vi "Robot Global Data.vi"() -> ()   [LabVIEW 2013]
doc: "This global VI can contain as many global variables as you need. Place a control on the panel, give it a good name. To read or write to it from a VI, drag the icon to the diagram of that VI. You can also drag from the project. Click on the node to change which global you access. You shouldn't have multiple locations writing to a global or it will cause a race-condition."
uses:
  <vilib>/Rock Robotics/WPI/DriverStation/WPI_DriverStationRobotMode2.ctl
  Drivetrain/Drivetrain Control.ctl
  Drivetrain/DT Mode.ctl
  Rollers/Roller Control.ctl
  Rollers/Roller Mode.ctl
  Common Code/Vision Packet.ctl
  Common Code/Goal Info.ctl
  Drivetrain/Arcade Drive Ref.ctl
  <vilib>/Rock Robotics/WPI/MotorControl/WPI_MotorControlDeviceRef.ctl
  <vilib>/Rock Robotics/SystemInterfaces/Typedef/FPGA_TypedefDigitalModule.ctl
  <vilib>/Rock Robotics/SystemInterfaces/DIO/FPGA_DIOPWMChannel.ctl
  <vilib>/Rock Robotics/WPI/PWM/WPI_PWMDeadband.ctl
  <vilib>/Rock Robotics/WPI/CAN/Jaguar/SubVIs/WPI_CANJaguar_ControlMode.ctl
  <vilib>/Rock Robotics/WPI/PWM/WPI_PWMTransform_ConPane.ctl
  Shooter/Shooter Manual Control.ctl
  Shooter/Shooter Command.ctl
  Drivetrain/Distance Drive Result.ctl
  Common Code/Dashboard UDP Packet.ctl
  Common Code/Dashboard UDP/Camera Controls.ctl
  Common Code/Dashboard UDP/Gyro Controls.ctl
  Common Code/Dashboard UDP/PID Params.ctl
  Common Code/Dashboard UDP/Encoder Controls.ctl
  Common Code/Dashboard UDP/Auto Shift Controls.ctl
  Common Code/Dashboard UDP/Auton Controls.ctl
  Common Code/Dashboard UDP/Shooter Controls.ctl
  Common Code/Dashboard UDP/Roller Controls.ctl
  Common Code/Vision Mode.ctl
  Common Code/Dashboard UDP/Fieldcentric Controls.ctl
  Common Code/Dashboard UDP/Roll Maneuver.ctl
  Drivetrain/Drivetrain Status.ctl
  Rollers/Roller Status.ctl
  Common Code/IR Logic State.ctl
  Shooter/Shooter Status.ctl
  Common Code/Shooter State.ctl
panel:
  out "Auton Enabled Time":u32
  out "Invert Halo":bool
  out "Halo Up Time":i32
  out "Halo":bool
  out "Manual Halo":bool
  out "Auto Halo":bool
  out "Shooter Wants Halo":bool
  out "Roller Wants Halo":bool
  out "100ms Loop Time":i32
  out "Auton File Display":string
  out "Auton Command Count":i32
  out "Auton Command":i32
  out "Shooter Status":T1
  out "Roller Status":T3
  out "Gyro Target":dbl
  out "Drivetrain Status":T5
  in  "Auton File":dbl
  out "UDP Packet":T7={"Camera"={"Camera/View Angle X"=66.5, "Camera/Goal Track Timeout"=120.0, "Camera/View Angle Y"=49.0, "Camera/Goal Exposure"=0.0, "Camera/Vision Receive Timeout"=120.0, "Camera/Offset 1"=-35.0, "Camera/Offset 2"=35.0}, "Gyro"={"Gyro/Angle Tolerance"=2.0, "Gyro/Steer Closeness Threshold"=10.0, "Steer PID"={"max"=0.8, "min"=-0.8, "P"=0.04, "I"=0.0, "D"=0.0}, "Steer Close PID"={"max"=0.7, "min"=-0.7, "P"=0.04, "I"=0.0, "D"=0.002}}, "Encoder"={"Encoders/Reset"=FALSE, "Encoders/Omni Constant"=0.002909, "Encoders/Omni Tick Constant"=1.0, "Encoders/Left Constant"=0.000546, "Encoders/Right Constant"=0.000546, "Encoders/Right Tick Constant"=1.0}, "Auto Shift"={"AutoShift/Upshift Throttle Accel"=-2.0, "AutoShift/Speed Threshold"=5.0, "AutoShift/Upshift Throttle"=0.8, "AutoShift/Upshift Accel"=0.5, "AutoShift/Downshift Accel"=-1.2, "AutoShift/Downshift Throttle"=0.15, "AutoShift/Delay"=1000.0, "AutoShift/Enabled"=TRUE}, "Auton"={"Auton/Left Shoot X-Coord"=-4.0, "Auton/Right Shoot X-Coord"=4.0, "DistDrive/Distance Stop Threshold"=0.25, "DistDrive/Max Stop Speed"=0.5, "Auton/Back Piston Time"=500.0, "Auton/Manual Hot"=FALSE, "Auton/Manual Hot Right"=FALSE, "Default X PID"={"max"=1.0, "min"=-1.0, "P"=0.36, "I"=0.0, "D"=0.0}, "Default Y PID"={"max"=1.0, "min"=-1.0, "P"=0.7, "I"=0.0, "D"=0.001}, "Half Over Delay"=4500.0}, "Drive/Ramp X"=500.0, "Drive/Ramp Y"=250.0, "Drive/Battery Cutoff"=6.0, "Pressure/Compressor Min Voltage"=7.0, "Pressure/Compressor Delay"=500.0, "Controller/Strafe Correction"=TRUE, "Shooter"={"Shooter/Reset Time"=500.0, "Shooter/Release Delay"=150.0, "Shooter/Pressure Steady Time"=0.0, "Shooter/Misfire Delay"=2000.0, "Shooter/Ball Settle Time"=500.0, "Shooter/Line IR Delay"=300.0, "Pressure/Upper PSI Time"=500.0, "Pressure/Lower PSI Time"=500.0, "Shooter/Punch Delay"=-150.0, "Shooter/Target Pressure"=43.0, "Pressure/Line B"=-57.077, "Pressure/Line M"=33.41, "Pressure/Shooter M"=33.41, "Pressure/Shooter B"=-57.077, "Halo Time"=150.0, "Soft Release Delay"=800.0, "Soft Unpin Delay"=250.0, "Soft Shoot Delay"=290.0, "Toss Release Time"=62.4}, "Rollers"={"Roller/Load IRs Verify Time"=150.0, "Roller/Center IR Latch Time"=500.0, "Roller/Speed Front"=1.0, "Roller/Speed Back"=0.6, "Roller/Entry Timeout"=750.0, "Roller/To Center Timeout"=2000.0, "Roller/Sustain Time"=5000.0, "Roller/Verify Center Time"=250.0}, "Abort"=FALSE, "Finish"=FALSE, "IR Halo Sustain Time"=0.0, "Disable Compressor"=FALSE, "Center Omni Drive Delay"=100, "Vision Mode"=enum."Normal", "Radius Throttle"=TRUE, "Fieldcentric"={"Relative Angle"=TRUE, "Point Robot"=FALSE, "X/Y ratio low"=0.75, "Steering Gain"=1.0, "Force Omni Down"=TRUE, "Enable"=TRUE, "X/Y ratio high"=0.5}, "Roll"={"X 1"=0.0, "Y 1"=1.0, "Y 2"=1.0, "X 2"=1.0, "Y 3"=1.0, "X 3"=0.0, "Time 1"=300, "Time 2"=1000, "Time 3"=0, "Angle Start"=0.0, "Angle End"=-180.0, "Angle Linearity"=1.0}, "Stick Deadband"=0.075}
  out "Distance Drive Result":T19
  out "Robot Direction":enum16{"Forward", "Backward"}(ring)
  out "Robot Orientation":enum16{"Away", "Towards"}(ring)
  out "LineJustCrossed":enum16{"None", "Blue", "Red"}(ring)
  out "Zone":enum16{"Blue", "White", "Red"}(ring)=enum."Red"
  out "Line Crossed?":bool
  out "Line Heading Towards":enum16{"Red", "Blue"}(ring)
  out "Last Shoot Begin Time":u32
  out "Goals Used":i32
  out "Hot Found":bool
  out "Shoot High Pressure":bool
  in  "Interrupt Negated":bool
  in  "Finish":bool
  in  "Abort":bool
  in  "Interrupt Condition":i32
  in  "Interrupt Index":i32
  in  "Interrupt Set":bool
  out "Gyro Calibrating":bool
  out "Recalibrate Gyro":refnum<k4>
  out "Last Shoot Time":u32
  out "Camera 2 Packet":T20
  out "Camera 2 Connected":bool
  out "Camera 1 Connected":bool
  in  "Shooter Control":T22
  out "Gyro in Range":bool
  in  "Roller Control":T24
  out "Find Ball?":bool
  in  "isQuietRun":bool
  out "isRightHot":bool
  out "Cam Search Enabled":bool
  in  "Vision UDP Connection":refnum<k16>
  in  "Selection controls":cluster{"Up":bool, "Down":bool}
  in  "FilesInAutonDir":i32
  out "Camera 1 Packet":T20
  out "Auto Array":dbl[][](array[numeric]) format="%0.3f"
  in  "Drivetrain Control":T26={"axis 1 (x)"=0.0, "axis 2 (y)"=0.0, "Mode"=enum."Manual", "heading target"=0.0, "steer axis"=0.0, "omni?"=FALSE, "Low Gear?"=FALSE, "distance target"={"x"=0.0, "y"=0.0}, "PID Params"={"X Dist"={"PID gains"={"proportional gain (Kc)"=1.0, "integral time (Ti, min)"=0.0, "derivative time (Td, min)"=0.0}, "output range"={"output high"=1.0, "output low"=-1.0}}, "Y Dist"={"PID gains"={"proportional gain (Kc)"=1.0, "integral time (Ti, min)"=0.0, "derivative time (Td, min)"=0.0}, "output range"={"output high"=1.0, "output low"=-1.0}}}, "Coast"=FALSE} {"PID Params"."Y Dist"."output range"."output low" format="%.2f"; "PID Params"."Y Dist"."output range"."output high" format="%.2f"; "PID Params"."Y Dist"."PID gains"."derivative time (Td, min)" format="%.3f"; "PID Params"."Y Dist"."PID gains"."integral time (Ti, min)" format="%.3f"; "PID Params"."Y Dist"."PID gains"."proportional gain (Kc)" format="%.3f"; "PID Params"."X Dist"."output range"."output low" format="%.2f"; "PID Params"."X Dist"."output range"."output high" format="%.2f"; "PID Params"."X Dist"."PID gains"."derivative time (Td, min)" format="%.3f"; "PID Params"."X Dist"."PID gains"."integral time (Ti, min)" format="%.3f"; "PID Params"."X Dist"."PID gains"."proportional gain (Kc)" format="%.3f"}
  in  "Robot Mode":T27
  out "Arcade Drive":T28
  # "Note: default values here are meaningless,\nSet default values in \"Load Preferences.vi\""
  # "Autonomous Stuff"
  # "Line"
  # "Shooter"
  # "Down"
  # "Up"
  # "Feet"
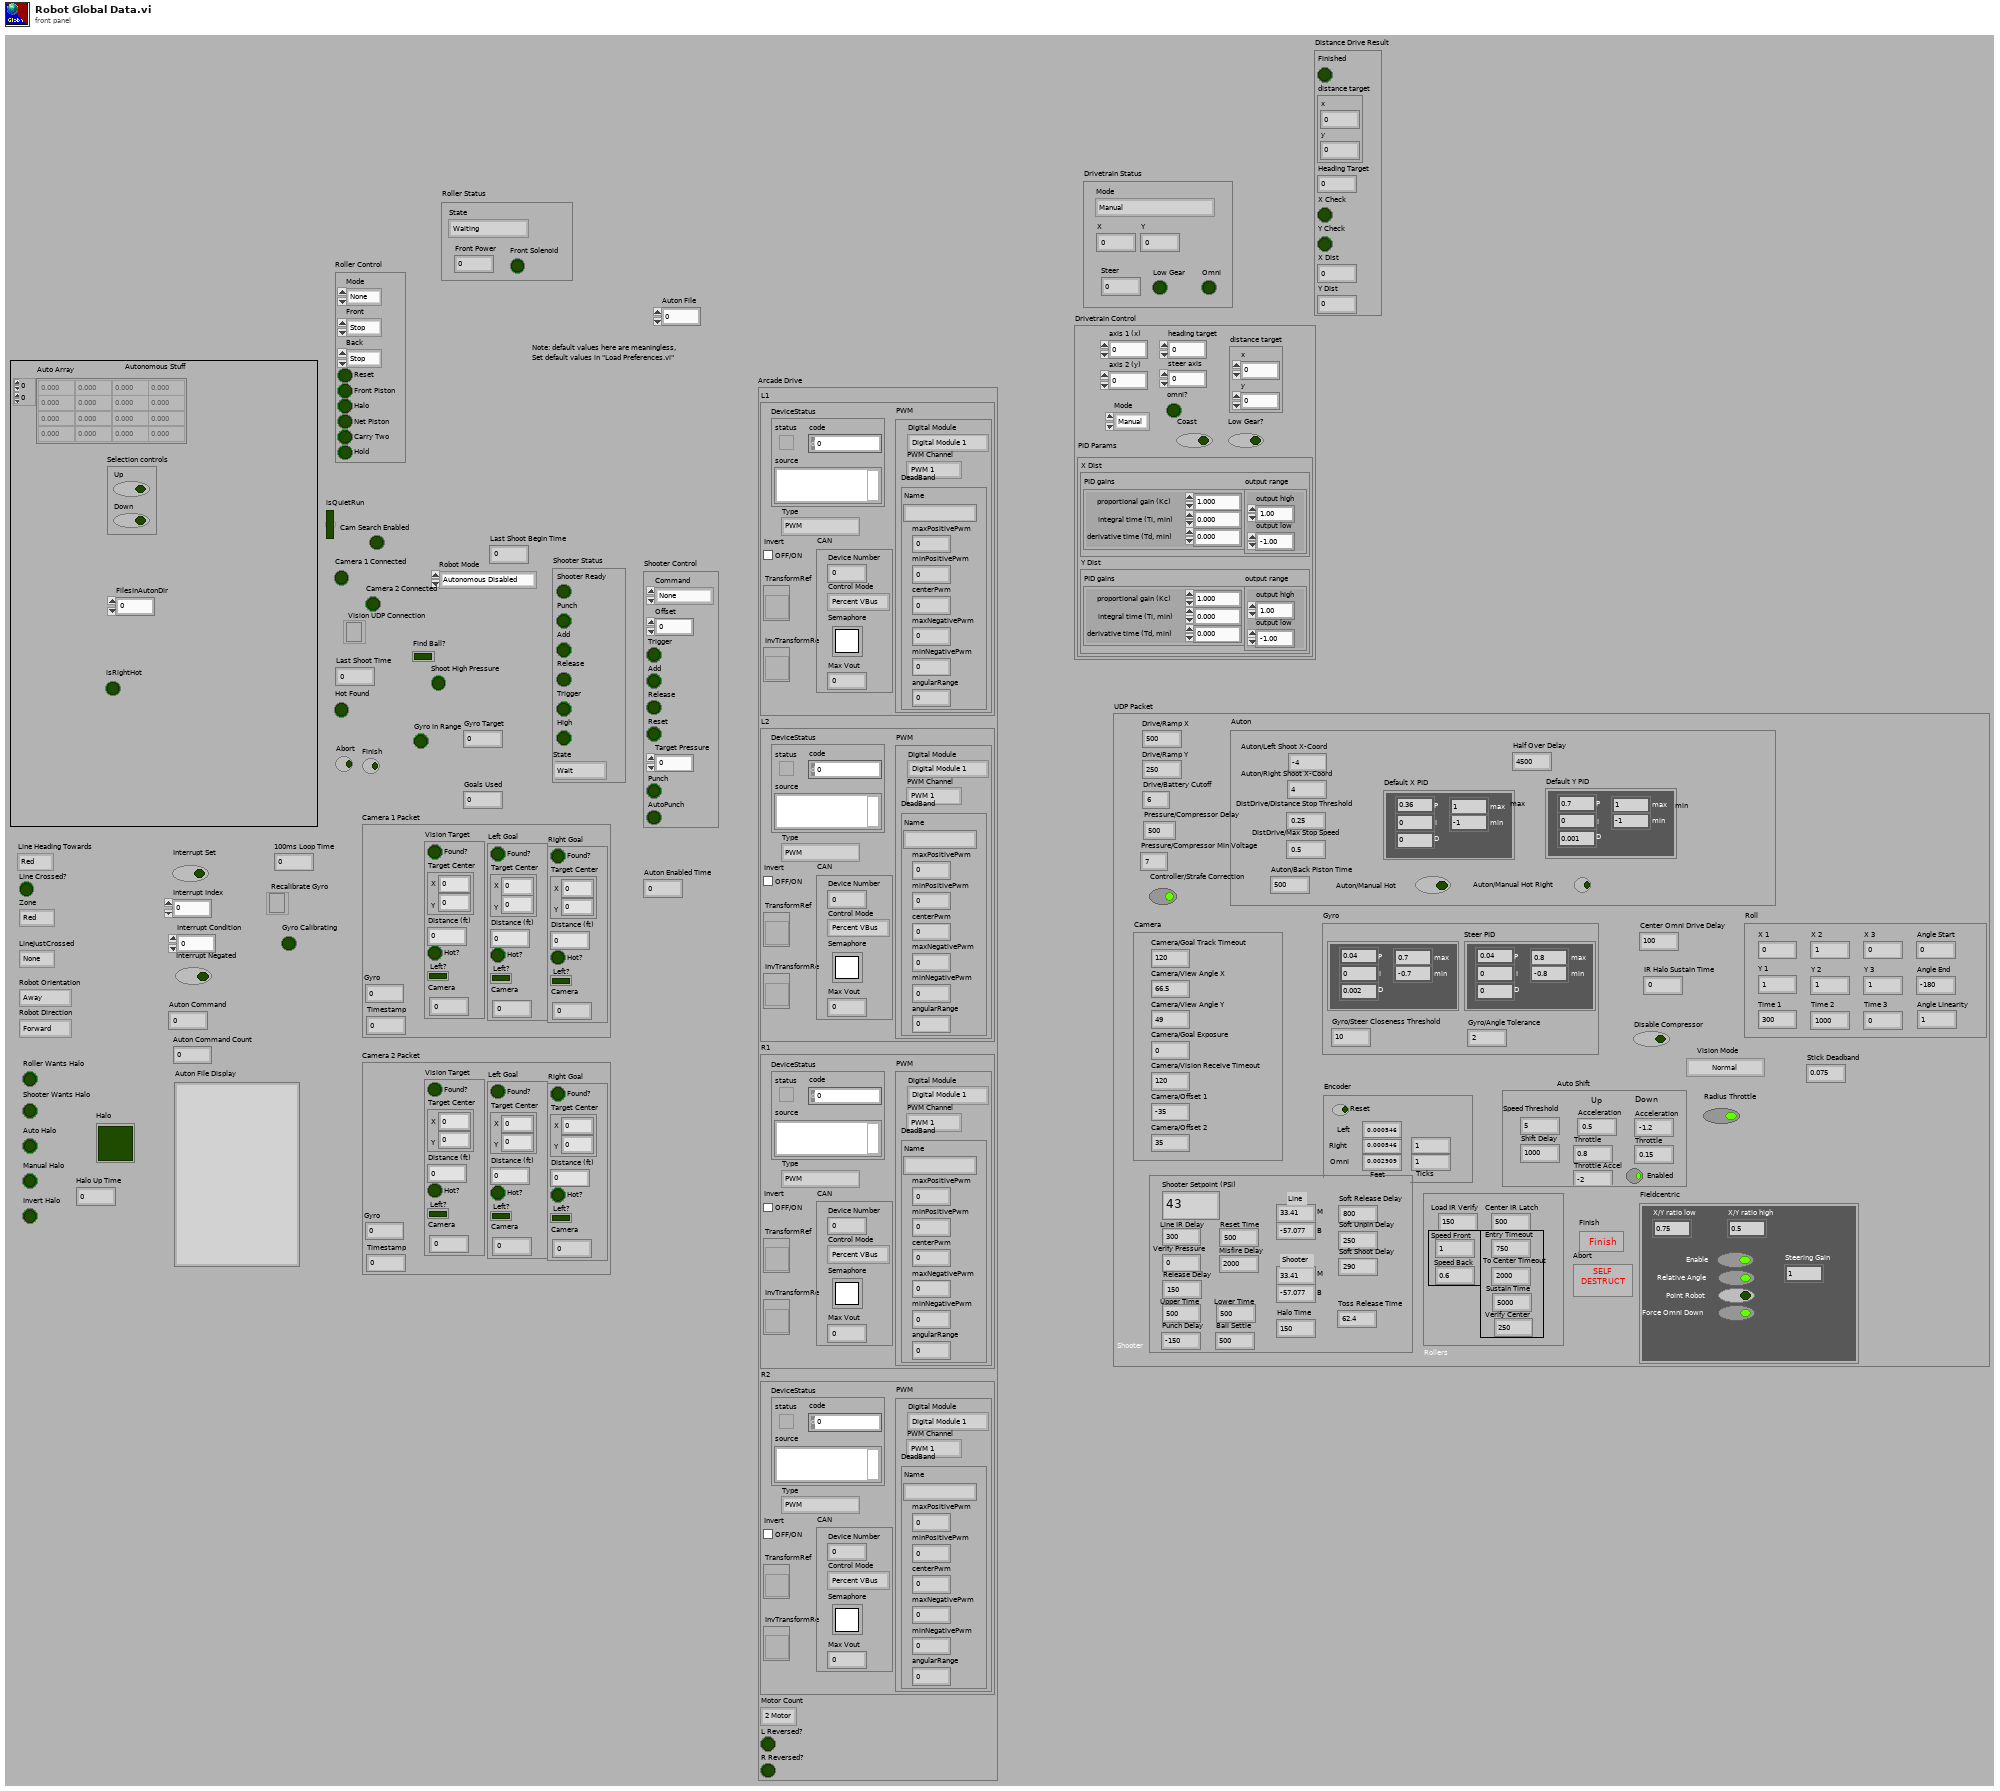
[diagram p1: front panel]
types:
  T1 = typedef "Shooter Status.ctl" = cluster{"Shooter Ready":bool, "Add":bool, "Punch":bool, "Release":bool, "Trigger":bool, "High":bool, "State":T2}
  T2 = typedef "Shooter State.ctl" = enum16{"Wait", "Fill Piston", "Lift Halo", "Trigger", "Reset", "Soft Release", "Soft Unpin", "Soft Refill", "Soft Shoot", "Toss Prep", "Toss Release"}
  T3 = typedef "Roller Status.ctl" = cluster{"State":T4, "Front Power":dbl, "Front Solenoid":bool}
  T4 = typedef "IR Logic State.ctl" = enum16{"Waiting", "Requested", "Loading", "Full", "Wait for Center", "Carry", "Full Carry", "Holding"}
  T5 = typedef "Drivetrain Status.ctl" = cluster{"Mode":T6, "X":dbl, "Y":dbl, "Steer":dbl, "Low Gear":bool, "Omni":bool}
  T6 = typedef "DT Mode.ctl" = enum16{"Manual", "Gyro Steer", "Distance Drive", "Fieldcentric", "Roll Maneuver", "Alt Roll Maneuver"}
  T7 = typedef "Dashboard UDP Packet.ctl" = cluster{"Camera":T8, "Gyro":T9, "Encoder":T11, "Auto Shift":T12, "Auton":T13, "Drive/Ramp X":dbl, "Drive/Ramp Y":dbl, "Drive/Battery Cutoff":dbl, "Pressure/Compressor Min Voltage":dbl, "Pressure/Compressor Delay":dbl, "Controller/Strafe Correction":bool, "Shooter":T14, "Rollers":T15, "Abort":bool, "Finish":bool, "IR Halo Sustain Time":dbl, "Disable Compressor":bool, "Center Omni Drive Delay":i32, "Vision Mode":T16, "Radius Throttle":bool, "Fieldcentric":T17, "Roll":T18, "Stick Deadband":dbl}
  T8 = typedef "Camera Controls.ctl" = cluster{"Camera/View Angle X":dbl, "Camera/Goal Track Timeout":dbl, "Camera/View Angle Y":dbl, "Camera/Goal Exposure":dbl, "Camera/Vision Receive Timeout":dbl, "Camera/Offset 1":dbl, "Camera/Offset 2":dbl}
  T9 = typedef "Gyro Controls.ctl" = cluster{"Gyro/Angle Tolerance":dbl, "Gyro/Steer Closeness Threshold":dbl, "Steer PID":T10, "Steer Close PID":T10}
  T10 = typedef "PID Params.ctl" = cluster{"max":dbl, "min":dbl, "P":dbl, "I":dbl, "D":dbl}
  T11 = typedef "Encoder Controls.ctl" = cluster{"Encoders/Reset":bool, "Encoders/Omni Constant":dbl, "Encoders/Omni Tick Constant":dbl, "Encoders/Left Constant":dbl, "Encoders/Right Constant":dbl, "Encoders/Right Tick Constant":dbl}
  T12 = typedef "Auto Shift Controls.ctl" = cluster{"AutoShift/Upshift Throttle Accel":dbl, "AutoShift/Speed Threshold":dbl, "AutoShift/Upshift Throttle":dbl, "AutoShift/Upshift Accel":dbl, "AutoShift/Downshift Accel":dbl, "AutoShift/Downshift Throttle":dbl, "AutoShift/Delay":dbl, "AutoShift/Enabled":bool}
  T13 = typedef "Auton Controls.ctl" = cluster{"Auton/Left Shoot X-Coord":dbl, "Auton/Right Shoot X-Coord":dbl, "DistDrive/Distance Stop Threshold":dbl, "DistDrive/Max Stop Speed":dbl, "Auton/Back Piston Time":dbl, "Auton/Manual Hot":bool, "Auton/Manual Hot Right":bool, "Default X PID":T10, "Default Y PID":T10, "Half Over Delay":dbl}
  T14 = typedef "Shooter Controls.ctl" = cluster{"Shooter/Reset Time":dbl, "Shooter/Release Delay":dbl, "Shooter/Pressure Steady Time":dbl, "Shooter/Misfire Delay":dbl, "Shooter/Ball Settle Time":dbl, "Shooter/Line IR Delay":dbl, "Pressure/Upper PSI Time":dbl, "Pressure/Lower PSI Time":dbl, "Shooter/Punch Delay":dbl, "Shooter/Target Pressure":dbl, "Pressure/Line B":dbl, "Pressure/Line M":dbl, "Pressure/Shooter M":dbl, "Pressure/Shooter B":dbl, "Halo Time":dbl, "Soft Release Delay":dbl, "Soft Unpin Delay":dbl, "Soft Shoot Delay":dbl, "Toss Release Time":dbl}
  T15 = typedef "Roller Controls.ctl" = cluster{"Roller/Load IRs Verify Time":dbl, "Roller/Center IR Latch Time":dbl, "Roller/Speed Front":dbl, "Roller/Speed Back":dbl, "Roller/Entry Timeout":dbl, "Roller/To Center Timeout":dbl, "Roller/Sustain Time":dbl, "Roller/Verify Center Time":dbl}
  T16 = typedef "Vision Mode.ctl" = enum16{"Normal", "Extreme Left", "Extreme Right"}
  T17 = typedef "Fieldcentric Controls.ctl" = cluster{"Relative Angle":bool, "Point Robot":bool, "X/Y ratio low":dbl, "Steering Gain":dbl, "Force Omni Down":bool, "Enable":bool, "X/Y ratio high":dbl}
  T18 = typedef "Roll Maneuver.ctl" = cluster{"X 1":dbl, "Y 1":dbl, "Y 2":dbl, "X 2":dbl, "Y 3":dbl, "X 3":dbl, "Time 1":i32, "Time 2":i32, "Time 3":i32, "Angle Start":dbl, "Angle End":dbl, "Angle Linearity":dbl}
  T19 = typedef "Distance Drive Result.ctl" = cluster{"Finished":bool, "distance target":cluster{"x":dbl, "y":dbl}, "Heading Target":dbl, "X Check":bool, "Y Check":bool, "X Dist":dbl, "Y Dist":dbl}
  T20 = typedef "Vision Packet.ctl" = cluster{"Gyro":dbl, "Vision Target":T21, "Timestamp":u32, "Left Goal":T21, "Right Goal":T21}
  T21 = typedef "Goal Info.ctl" = cluster{"Found?":bool, "Target Center":cluster{"X":dbl, "Y":dbl}, "Distance (ft)":dbl, "Hot?":bool, "Left?":bool, "Camera":i16}
  T22 = typedef "Shooter Manual Control.ctl" = cluster{"Command":T23, "Offset":dbl, "Trigger":bool, "Add":bool, "Release":bool, "Reset":bool, "Target Pressure":dbl, "Punch":bool, "AutoPunch":bool}
  T23 = typedef "Shooter Command.ctl" = enum16{"None", "Warmup", "Shoot", "Line Shoot", "Soft Shoot", "Toss"}
  T24 = typedef "Roller Control.ctl" = cluster{"Mode":T25, "Front":enum16{"Stop", "Forward", "Reverse"}, "Back":enum16{"Stop", "Forward", "Reverse"}, "Reset":bool, "Front Piston":bool, "Halo":bool, "Net Piston":bool, "Carry Two":bool, "Hold":bool}
  T25 = typedef "Roller Mode.ctl" = enum16{"None", "Front", "Back", "Both", "Manual"}
  T26 = typedef "Drivetrain Control.ctl" = cluster{"axis 1 (x)":dbl, "axis 2 (y)":dbl, "Mode":T6, "heading target":dbl, "steer axis":dbl, "omni?":bool, "Low Gear?":bool, "distance target":cluster{"x":dbl, "y":dbl}, "PID Params":cluster{"X Dist":cluster{"PID gains":cluster{"proportional gain (Kc)":dbl, "integral time (Ti, min)":dbl, "derivative time (Td, min)":dbl}, "output range":cluster{"output high":dbl, "output low":dbl}}, "Y Dist":cluster{"PID gains":cluster{"proportional gain (Kc)":dbl, "integral time (Ti, min)":dbl, "derivative time (Td, min)":dbl}, "output range":cluster{"output high":dbl, "output low":dbl}}}, "Coast":bool}
  T27 = typedef "WPI_DriverStationRobotMode2.ctl" = enum16{"Autonomous Disabled", "Autonomous Enabled", "Teleop Disabled", "Teleop Enabled", "Timeout", "Finish", "Test Disabled", "Test Enabled"}
  T28 = typedef "Arcade Drive Ref.ctl" = cluster{"L1":T29, "L2":T29, "R1":T29, "R2":T29, "Motor Count":enum16{"2 Motor", "4 Motor"}, "L Reversed?":bool, "R Reversed?":bool}
  T29 = typedef "WPI_MotorControlDeviceRef.ctl" = cluster{"DeviceStatus":errorcluster, "Type":enum16{"PWM", "CAN"}, "PWM":cluster{"Digital Module":T30, "PWM Channel":T31, "DeadBand":T32}, "CAN":cluster{"Device Number":u8, "Control Mode":T33, "Semaphore":T34, "Max Vout":dbl}, "Invert":bool, "TransformRef":T35, "InvTransformRef":T35}
  T30 = typedef "FPGA_TypedefDigitalModule.ctl" = enum16{"Digital Module 1", "Digital Module 2"}
  T31 = typedef "FPGA_DIOPWMChannel.ctl" = enum8{"PWM 1", "PWM 2", "PWM 3", "PWM 4", "PWM 5", "PWM 6", "PWM 7", "PWM 8", "PWM 9", "PWM 10", "Invalid"}
  T32 = typedef "WPI_PWMDeadband.ctl" = cluster{"Name":string, "maxPositivePwm":i32, "minPositivePwm":i32, "centerPwm":i32, "maxNegativePwm":i32, "minNegativePwm":i32, "angularRange":u16}
  T33 = typedef "WPI_CANJaguar_ControlMode.ctl" = enum8{"Percent VBus", "Current", "Speed", "Position", "Voltage"}
  T34 = typedef "Semaphore RefNum" = refnum<k1>
  T35 = typedef "WPI_PWMTransform_ConPane.ctl" = refnum<vi>
diagram:
